vi "Read.EngineData.vi"(8 "error in":errorcluster, 11 "Read in":refnum<class "Read.lvclass">) -> (0 "error out":errorcluster, 3 "Read out":refnum<class "Read.lvclass">)   [LabVIEW 2024, in "VS Plugin Inline Async API.lvlib" / "Read.lvclass"]
uses:
  Read.lvclass
  Read.lvclass/Read.ctl
  VS Engine Interface/VS Engine Interface.lvclass
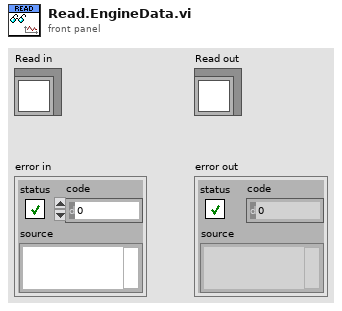
[diagram p1: front panel]
types:
  T1 = typedef "Custom Device API.lvlib/Block Data Reference.ctl" = cluster{"Data Reference":T2, "Offset":u64, "Length":u64}
  T2 = typedef "Custom Device API.lvlib/Data Reference.ctl" = i32
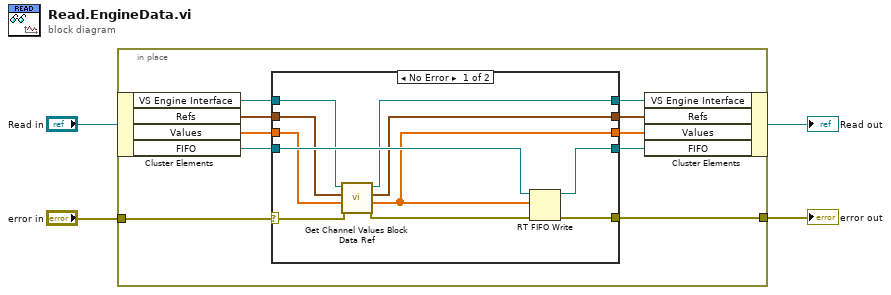
[diagram p0: block diagram]
diagram:
  n1 = in-place {
    in-place-border: [w14] -> w3
    in-place-border: "error in" -> [w13]
    n2 = in-place-cluster #1("Read in") -> ("VS Engine Interface"=w6:refnum<class "VS Engine Interface.lvclass">, "Refs"=w12:T1[], "Values"=w10:dbl[], "FIFO"=w8:refnum<k33>)
    n3 = case shown="No Error" w13 {
      selector: w13 -> [w24 w30]
      tunnel: [w25 w30] -> w14
      tunnel: [w17 w28] -> w9
      tunnel: w12 -> [w20 w29]
      tunnel: [w19 w29] -> w11
      tunnel: w10 -> [w18 w28]
      tunnel: w8 -> [w22 w27]
      tunnel: [w21 w27] -> w7
      tunnel: w6 -> [w16 w26]
      tunnel: [w15 w26] -> w5
      frame No Error {
        n4 = call-dynamic "Get Channel Values Block Data Ref.vi"("error in"=w24, "Values Array in"=w18, "Block Data Ref"=w20, "VS Engine Interface in"=w16) -> ("error out"=w23:errorcluster, "Values Array out"=w17:dbl[], "Block Data Ref dup"=w19:T1[], "VS Engine Interface out"=w15:refnum<class "VS Engine Interface.lvclass">)  [unwired: 4 in]
        n5 = RT FIFO Write(0:w22, 1:w17, 3:w23) -> (8:w21:refnum<k33>, 11:w25:errorcluster)  [unwired: 2 in, 2 out]
      }
      frame Error {
      }
    }
    n6 = in-place-cluster #1("VS Engine Interface"=w5, "Refs"=w11, "Values"=w9, "FIFO"=w7) -> (→"Read out":refnum<class "Read.lvclass">)
  }
  "error out" <- w3
